vi "Parse BOM Raw Data Row.vi"(8 "error in (no error)":errorcluster, 11 "BOM Table Row JSON":string) -> (0 "error out":errorcluster, 3 "BOM Table Raw Items":T1)   [LabVIEW 2018]
uses:
  TypeDef/BOM Table Raw Items.ctl
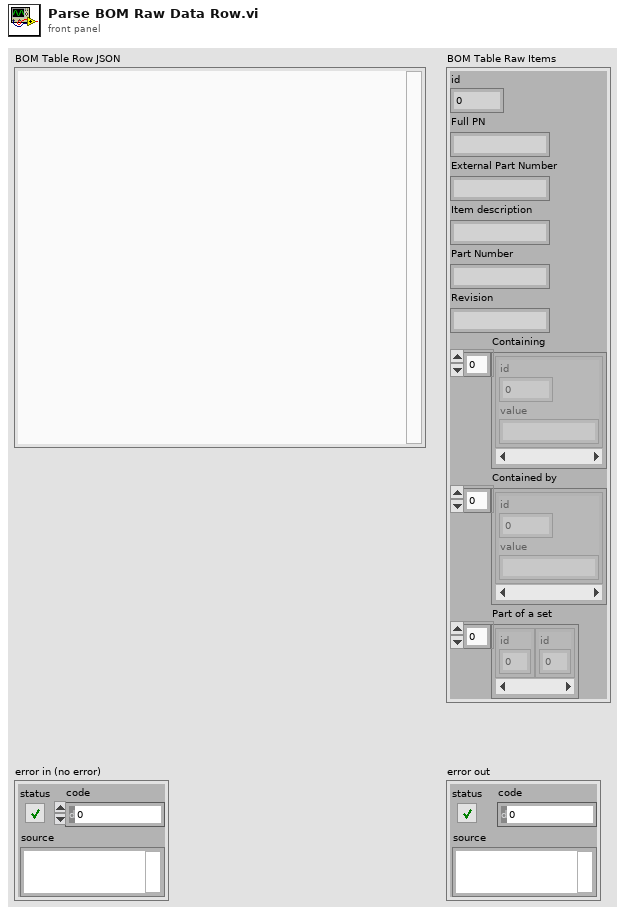
[diagram p1: front panel]
types:
  T1 = typedef "BOM Table Raw Items.ctl" = cluster{"id":i32, "Full PN":string, "External Part Number":string, "Item description":string, "Part Number":string, "Revision":string, "Containing":cluster{"id":i32, "value":string}[], "Contained by":cluster{"id":i32, "value":string}[], "Part of a set":cluster{"id":i32}[]}
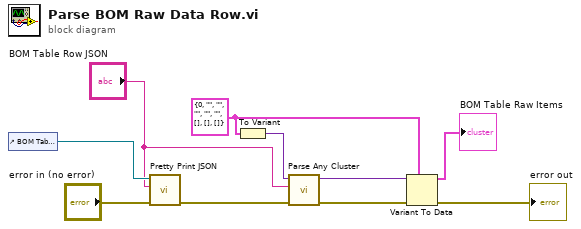
[diagram p0: block diagram]
diagram:
  w10 = T1 {"id"=0, "Full PN"="", "External Part Number"="", "Item description"="", "Part Number"="", "Revision"="", "Containing"=[], "Contained by"=[], "Part of a set"=[]}
  n1 = control-ref of="BOM Table Row JSON"() -> (w2:refnum<vi>)
  n2 = call "Pretty Print JSON.vi"("error in (no error)"="error in (no error)", "JSON in"="BOM Table Row JSON", "String in"=w2) -> ("error out"=w3:errorcluster)  [unwired: 8 in]
  n3 = To Variant(anything=w10) -> (Variant=w7:variant)
  n4 = call "Parse Any Cluster.vi"("error in (no error)"=w3, "JSON In"="BOM Table Row JSON", "Cluster in"=w7) -> ("error out"=w5:errorcluster, "Cluster out"=w6:variant)  [unwired: 7 in]
  n5 = Variant To Data(error in=w5, type=w10, Variant=w6) -> (data=→"BOM Table Raw Items":T1, error out=→"error out":errorcluster)
